vi "6-1.vi"   [LabVIEW 2017]
types:
  T1 = enum16{"open", "replace", "create", "open or create", "replace or create", "replace or create with confirmation"}
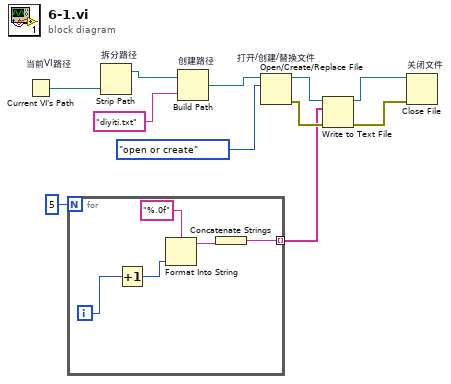
[diagram p0: block diagram]
diagram:
  n1 = Current VI's Path "当前VI路径"() -> (path=w11:path)
  n2 = for {
    N: 5 -> [_]
    tunnel: [w13] -> w1 mode=indexing
    i -> [w16]
    n3 = Increment(x=w16) -> (x+1=w15:i32)
    n4 = Format Into String(format string="%.0f" ("格式字符串"), w15) -> (resulting string=w14:string)  [unwired: 2 in, 1 out]
    n5 = Concatenate Strings(w14) -> (w13:string)
  }
  n6 = Strip Path "拆分路径"(path=w11) -> (stripped path=w10:path)  [unwired: 1 out]
  n7 = Build Path "创建路径"(base path=w10, name or relative path="diyiti.txt" ("名称或相对路径")) -> (appended path=w9:path)
  n8 = Open/Create/Replace File "打开/创建/替换文件"(file path (use dialog)=w9, operation (0:open)=T1."open or create" ("操作(0:open)")) -> (refnum out=w7:refnum<file>, error out=w3:errorcluster)  [unwired: 4 in, 1 out]
  n9 = Write to Text File(file (use dialog)=w7, text=w1, error in=w3) -> (refnum out=w8:refnum<file>, error out=w2:errorcluster)  [unwired: 1 in, 1 out]
  n10 = Close File "关闭文件"(refnum=w8, error in=w2) -> ()  [unwired: 2 out]
